vi "niLvFpga_Run_cRIO-9048.vi"(0 "session in":u32, 5 "Wait Until Done (F)":bool, 7 "control register address":u32 format="%.0x", 11 "error in":errorcluster) -> (4 "session out":u32, 15 "error out":errorcluster)   [LabVIEW 2020]
uses:
  <vilib>/rvi/interface/common/niFpgaWaitOnOcc.vi
  NiFpgaLv.dll
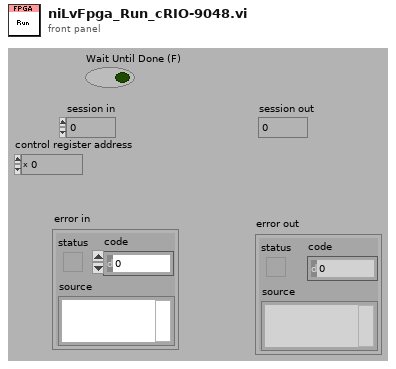
[diagram p1: front panel]
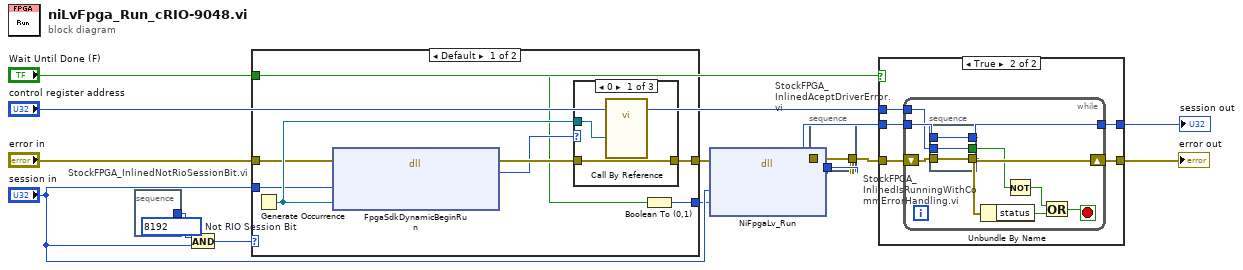
[diagram p0: block diagram]
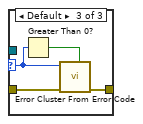
[diagram p4: hidden frame]
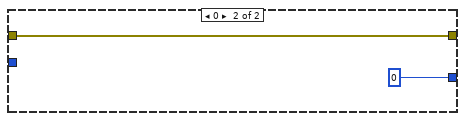
[diagram p5: hidden frame]
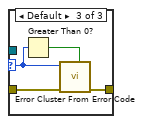
[diagram p9: hidden frame]
diagram:
  n1 = stacked-sequence "StockFPGA_InlinedNotRioSessionBit.vi" {
    tunnel: [w15] -> w7
    frame #0 {
      w15 = u32 8192  # Not RIO Session Bit
    }
  }
  n2 = And(x=w7, y="session in") -> (x .and. y?=w3:u32)
  n3 = case shown="Default" w3 {
    tunnel: "error in" -> [w20 w32]
    tunnel: [w19 w32] -> w5
    tunnel: "session in" -> [w18 _]
    tunnel: "Wait Until Done (F)" -> [w17 _]
    tunnel: [w16 u32 0 ("attribute")] -> w1
    frame Default {
      n4 = Generate Occurrence() -> (w23:refnum<k4>)
      n5 = dll-call lib="LabVIEW" fn="FpgaSdkDynamicBeginRun"(error in=w20, "session"=w18, "occurrence"=w23) -> (error out=w22:errorcluster, "status"=w21:i32)  [unwired: 4 in, 1 out]
      n6 = case shown="0" w21 {
        selector: w21 -> [_ _ w27]
        tunnel: [w25 w26 w29] -> w19
        tunnel: w22 -> [w25 w26 w30]
        tunnel: w23 -> [w24 _ _]
        frame 0 {
          n7 = call-by-ref "?"("occurrence"=w24) -> ()  [unwired: 16 in, 3 out]
        }
        frame -61167 {
          # "emulation case intentionally ignoring error"
        }
        frame Default {
          n8 = Greater Than 0?(x=w27) -> (x > 0?=w28:bool)
          n9 = call <vilib>:"Error Cluster From Error Code.vi"("is warning? (False)"=w28, "error in (no error)"=w30, "error code (0)"=w27) -> ("error out"=w29:errorcluster)  [unwired: 6 in]
        }
      }
      n10 = Boolean To (0,1)(Boolean=w17) -> (0, 1=w16:i16)
    }
    frame 0 {
    }
  }
  n11 = dll-call lib="NiFpgaLv.*" fn="NiFpgaLv_Run" label="niLvFpgaRun"(error in=w5, "sessionID"="session in", "attribute"=w1) -> (error out=w12:errorcluster, "status"=w11:i32, "sessionID"=w14:u32)  [unwired: 3 in, 1 out]
  n12 = stacked-sequence "StockFPGA_InlinedAceptDriverError.vi" {
    tunnel: w12 -> [w33]
    tunnel: w11 -> [w35]
    tunnel: [w34] -> w9
    frame #0 {
      n13 = case shown="Default" w35 {
        selector: w35 -> [_ w37]
        tunnel: [w36 w39] -> w34
        tunnel: w33 -> [w36 w40]
        frame 0 {
        }
        frame Default {
          n14 = Greater Than 0?(x=w37) -> (x > 0?=w38:bool)
          n15 = call <vilib>:"Error Cluster From Error Code.vi"("is warning? (False)"=w38, "error in (no error)"=w40, "error code (0)"=w37) -> ("error out"=w39:errorcluster)  [unwired: 6 in]
        }
      }
    }
  }
  n16 = case shown="True" "Wait Until Done (F)" {
    tunnel: w14 -> [w42 w47]
    tunnel: [w41 w46] -> w10
    tunnel: "control register address" -> [_ w45]
    tunnel: w9 -> [w41 w44]
    tunnel: [w42 w43] -> w8
    frame False {
    }
    frame True {
      n17 = while {
        tunnel: w47 -> [w51]
        shift-right: [w52] -> w46
        shift-left: w44 -> [w53]
        tunnel: w45 -> [w50]
        tunnel: [w49] -> w43
        stop <- w54 stop-if-true
        n18 = stacked-sequence "StockFPGA_InlinedIsRunningWithCommErrorHandling.vi" {
          tunnel: w51 -> [w61]
          tunnel: [w61] -> w49
          tunnel: w50 -> [w59]
          tunnel: [w60] -> w48
          tunnel: w53 -> [w57]
          tunnel: [w58] -> w52
          frame #0 {
            n19 = case shown="No Error" w57 {
              selector: w57 -> [w66 w113]
              tunnel: w61 -> [w68 _]
              tunnel: [w72 w113] -> w58
              tunnel: w59 -> [w67 _]
              tunnel: [w64 _] -> w60
              frame No Error {
                w76 = u32 16  # comm timeout bit
                # "If enable in is true and\nenable out is false, the vi\nis running."
                n20 = stacked-sequence "niLvFpga_Read32_cRIO-9048.vi" {
                  tunnel: w68 -> [w87]
                  tunnel: [w82] -> _
                  tunnel: w67 -> [w88]
                  tunnel: [w78] -> w65
                  tunnel: w66 -> [w85]
                  tunnel: [w81] -> w62
                  frame #0 {
                    n21 = stacked-sequence "StockFPGA_InlinedNotRioSessionBit.vi" {
                      tunnel: [w97] -> w84
                      frame #0 {
                        w97 = u32 8192  # Not RIO Session Bit
                      }
                    }
                    n22 = And(x=w84, y=w87) -> (x .and. y?=w83:u32)
                    n23 = case shown="Default" w83 {
                      tunnel: w85 -> [w103 w112]
                      tunnel: [w104 w112] -> w86
                      tunnel: w87 -> [w100 _]
                      tunnel: w88 -> [w99 _]
                      frame Default {
                        n24 = Generate Occurrence() -> (w101:refnum<k4>)
                        n25 = dll-call lib="LabVIEW" fn="FpgaSdkDynamicBeginRead"(error in=w103, "session"=w100, "occurrence"=w101, "index"=w99) -> (error out=w102:errorcluster, "status"=w98:i32)  [unwired: 5 in, 1 out]
                        n26 = case shown="0" w98 {
                          selector: w98 -> [_ _ w109]
                          tunnel: [w106 w107 w111] -> w104
                          tunnel: w101 -> [w105 _ _]
                          tunnel: w102 -> [w106 w107 w108]
                          frame 0 {
                            n27 = call-by-ref "?"("occurrence"=w105) -> ()  [unwired: 16 in, 3 out]
                          }
                          frame -61167 {
                            # "emulation case intentionally ignoring error"
                          }
                          frame Default {
                            n28 = Greater Than 0?(x=w109) -> (x > 0?=w110:bool)
                            n29 = call <vilib>:"Error Cluster From Error Code.vi"("is warning? (False)"=w110, "error in (no error)"=w108, "error code (0)"=w109) -> ("error out"=w111:errorcluster)  [unwired: 6 in]
                          }
                        }
                      }
                      frame 0 {
                      }
                    }
                    n30 = dll-call lib="NiFpgaLv.*" fn="NiFpgaLv_Read32" label="niLvFpgaRead32"(error in=w86, "session"=w87, "address"=w88) -> (error out=w79:errorcluster, "status"=w80:i32, "session"=w82:u32, "value"=w78:u32)  [unwired: 4 in, 1 out]
                    n31 = stacked-sequence "StockFPGA_InlinedAceptDriverError.vi" {
                      tunnel: w79 -> [w89]
                      tunnel: w80 -> [w91]
                      tunnel: [w90] -> w81
                      frame #0 {
                        n32 = case shown="Default" w91 {
                          selector: w91 -> [_ w93]
                          tunnel: [w92 w95] -> w90
                          tunnel: w89 -> [w92 w96]
                          frame 0 {
                          }
                          frame Default {
                            n33 = Greater Than 0?(x=w93) -> (x > 0?=w94:bool)
                            n34 = call <vilib>:"Error Cluster From Error Code.vi"("is warning? (False)"=w94, "error in (no error)"=w96, "error code (0)"=w93) -> ("error out"=w95:errorcluster)  [unwired: 6 in]
                          }
                        }
                      }
                    }
                  }
                }
                n35 = And(x=w65, y=u32 3) -> (x .and. y?=w70:u32)
                n36 = Equal?(x=w70, y=u32 2) -> (x = y?=w64:bool)
                n37 = And(x=w65, y=w76) -> (x .and. y?=w77:u32)
                n38 = Equal?(x=w77, y=w76) -> (x = y?=w63:bool)
                n39 = Select(t=-61046 ("error code (0)"), s=w63, f=0 ("error code (0)")) -> (s? t:f=w73:i32)
                n40 = call <vilib>:"Error Cluster From Error Code.vi"("error in (no error)"=w62, "error code (0)"=w73) -> ("error out"=w72:errorcluster)  [unwired: 1 in, 6 out]
              }
              frame Error {
              }
            }
          }
        }
        n41 = Unbundle By Name(w52) -> ("status"=w56:bool)
        n42 = Not(x=w48) -> (.not. x?=w55:bool)
        n43 = Or(x=w55, y=w56) -> (x .or. y?=w54:bool)
      }
    }
  }
  "error out" <- w10
  "session out" <- w8
